vi "Dashboard Main.vi"() -> ()   [LabVIEW 2016]
uses:
  <vilib>/event_ctls.llb/eventvkey.ctl
  <vilib>/Rock Robotics/WPI/Dashboard/WPI_DashboardLogging Global.vi
  <vilib>/Utility/miscctls.llb/LVRowAndColumnTypeDef.ctl
  <vilib>/Rock Robotics/Network Tables/NT Read Numeric Array.vi
panel:
  in  "DB/Slider 0":dbl(slide) caption="Trim" scale=0.0..1.0
  in  "DB/Button 0":bool caption="Enable\nOverdrive"
  in  "DB/Slider 4":dbl(slide) caption="Aiming Aides" scale=0.0..5.0
  in  "Camera Settings Right":T1={"Frame Rate"=30, "Compression"=30, "Size"=1, "DB Camera Config"=FALSE} {"Frame Rate" scale=1.0..30.0; "Compression" scale=100.0..-1.0; "Size" items=["640x480", "320x240", "160x120"]}
  in  "Camera Name Right":string(combo)="No Camera Selection"
  out "Camera Info":cluster{"Mbps LED":bool, "Mbps":dbl, "fps":dbl} {"fps" format="%#.1g"; "Mbps" format="%#.1g"}
  in  "Camera Settings":T1={"Frame Rate"=30, "Compression"=30, "Size"=1, "DB Camera Config"=FALSE} {"Frame Rate" scale=1.0..30.0; "Compression" scale=100.0..-1.0; "Size" items=["640x480", "320x240", "160x120"]}
  in  "TCP":refnum<k5>
  in  "Rec Mode":enum32{"Stop", "Record", "Playback"}(radio)
  out "Robot IP":string
  out "Image Message":string="Timeout in Camera Communications"
  in  "Dashboard Tab":T2(tab)
  in  "Trim":dbl(slide) scale=0.0..1.0
  in  "Overdrive Enabled?":bool
  in  "Select Auto":string(combo)="Select Autonomous ..."
  out "NT Connection":bool
  out "MotorChart R":cluster{"Numeric":dbl, "Numeric":dbl}(graph)
  out "MotorChart L":cluster{"Numeric":dbl, "Numeric":dbl}(graph)
  out "MotorSliders R":cluster{"MotorSlide1":dbl, "MotorSlide2":dbl} {"MotorSlide2" scale=-1.0..1.0 scale format="%#_2e"; "MotorSlide1" scale=-1.0..1.0 scale format="%#_2e"}
  out "MotorSliders L":cluster{"MotorSlide1":dbl, "MotorSlide2":dbl} {"MotorSlide2" scale=-1.0..1.0 scale format="%#_2e"; "MotorSlide1" scale=-1.0..1.0 scale format="%#_2e"}
  out "Gyro":dbl(knob) scale=0.0..360.0
  out "JS1 Z":dbl(slide) scale=-1.0..1.0 scale format="%#_2e"
  out "JS1 Graph":cluster{"X":dbl, "Y":dbl}[](graph)
  out "JS1 Buttons":T3
  out "JS2 Z":dbl(slide) scale=-1.0..1.0 scale format="%#_2e"
  out "JS2 Graph":cluster{"X":dbl, "Y":dbl}[](graph)
  out "JS2 Buttons":T3
  out "Mode":T4(ring)=enum."Auto Disabled"
  out "Camera Image Right":T5(plugin-control)
  in  "DB/String 9":string
  in  "DB/String 8":string
  in  "DB/String 7":string
  in  "DB/String 6":string
  in  "DB/String 5":string
  in  "DB/String 4":string
  in  "DB/String 3":string
  in  "DB/String 2":string
  in  "DB/String 1":string
  in  "DB/String 0":string
  in  "DB/Slider 1":dbl(slide) caption="Aiming Aides" scale=0.0..5.0
  in  "DB/Slider 2":dbl(slide) scale=0.0..5.0
  in  "DB/Slider 3":dbl(slide) scale=0.0..5.0
  out "DB/LED 3":bool
  out "DB/LED 2":bool
  out "DB/LED 1":bool
  out "DB/LED 0":bool caption="Throttle"
  in  "DB/Button 3":bool
  in  "DB/Button 2":bool
  in  "DB/Button 1":bool
  out "Calibrated?":bool
  in  "Reset Angle":bool
  in  "Test Slider":dbl(slide) scale=0.0..100.0 scale format="%#_3g"
  in  "On/Off":bool caption="Solenoid"
  in  "Test Name":u16(ring) items=["Select the test to run..."]
  in  "Test Tree":string(tree)
  in  "Motor":cluster{"Value":dbl, "Enable":bool} {"Value" scale=-1.0..1.0 scale format="%#_3g"}
  out "Progress":T6 {"Test Progress" scale=0.0..100.0}
  in  "Rev/Fwd":cluster{"Forward":bool, "Reverse":bool}
  in  "Test Ring":u16(ring) items=["Monochrome", "Color"]
  out "Cmd Status":string
  in  "Execute Command":bool
  in  "Command Params":string[][](table)
  in  "Command Selection":i32(listbox)
  in  "CheckList":i32(listbox)
  out "Tree":string(tree)
  out "Camera Image":T5(plugin-control)
  in  "Camera Name":string(combo)="No Camera Selection"
  # "HW"
  # "HW"
  # "Joysticks"
  # "Drive Motors"
  # "Front"
  # "Right"
  # "Left"
  # "Back"
  # "This tab is a great place for autonomous settings and robot-specific values.\nPlace controls and indicators inside this tab and match name to\nDashboard Variables on robot. You can also delete this comment."
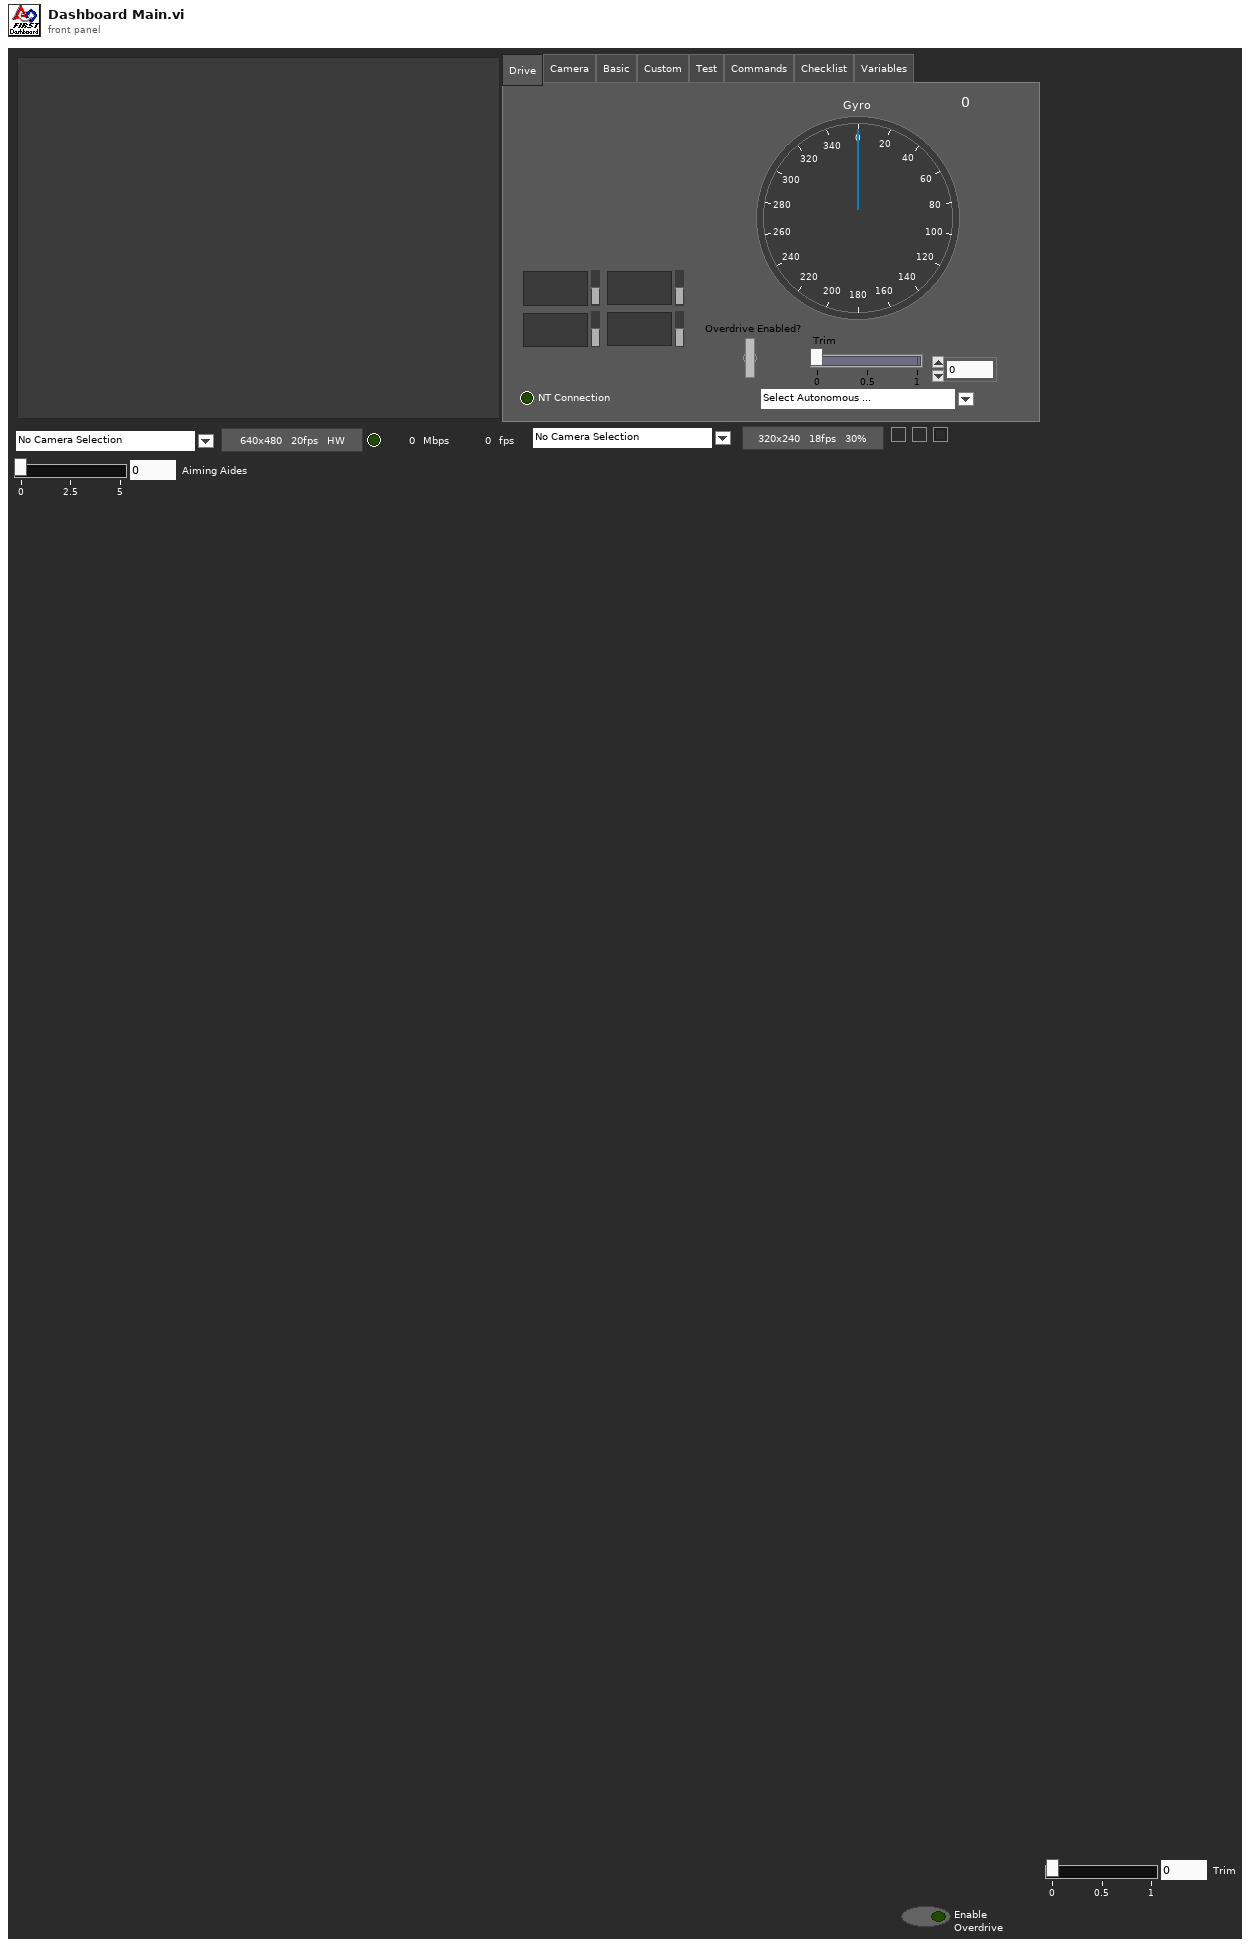
[diagram p1: front panel]
types:
  T1 = cluster{"Frame Rate":i32, "Compression":i32, "Size":u16, "DB Camera Config":bool}
  T2 = enum32{"Drive", "Camera", "Basic", "Custom", "Test", "Commands", "Checklist", "Variables"}
  T3 = cluster{bool, bool, bool, bool, bool, bool, bool, bool, bool, bool, bool, bool}
  T4 = enum8{"Tele-Op Disabled", "Tele-Op Enabled", "Auto Disabled", "Auto Enabled", "Test Disabled", "Test Enabled", "Disconnected", "No Code", "E-Stop"}
  T5 = typedef "IMAQ Image.ctl" = refnum<image>
  T6 = cluster{"Test Progress":u8, "Test Progress Text":string}
  T7 = typedef "Image Type" = u32
  T8 = cluster{"IDs":cluster{"RPC field ID":u16, "Unique ID":u16}, "String":string}
  T9 = enum32{"Drive", "Basic", "Custom", "Test", "Checklist", "Variables"}
  T10 = cluster{"Error Strings":string, "Disable Counts":cluster{u16, u16}, "Rail Faults":cluster{u16, u16, u16}, "Robot IP":string, "DB Mode":u8, "Event Info":cluster{"Name":string, "Type":u8, "Number":u16, "Replay":u8}}
  T11 = cluster{"Storage":cluster{"Disk Free":u64, "RAM Block":u32, "RAM free":u32}, "CPU Utilization":cluster{"CPU % ISR":sgl, "CPU % Time Crit":sgl, "CPU % Timed Str":sgl, "CPU % High":sgl, "CPU % Above":sgl, "CPU % Normal":sgl, "CPU % Low":sgl}, "CAN":cluster{"% Bus Utilization":sgl, "Bus Off Cnt":u32, "TX_FIFO Full Cnt":u32, "Receive Error Cnt":u8, "Transmit Error Cnt":u8}, "HID":cluster{"HID Outputs":u32, "Rumble Low":u16, "Rumble High":u16}[]}
  T12 = cluster{"Status bits":cluster{"Test Mode":bool, "Autonomous":bool, "Enabled":bool, "Code Start":bool, "Brownout":bool, "Reserved 2":bool, "Reserved 3":bool, "E-Stop":bool}, "Code Trace":cluster{"Disabled":bool, "TeleOp":bool, "Auto":bool, "Test":bool}, "Controller Type":enum16{"unknown", "cRIO", "roboRio"}, "Code?":enum16{"unknown", "noCode", "code"}, "Battery V":dbl}
  T13 = cluster{"Control Bits":cluster{"TestMode":bool, "Autonomous":bool, "Enabled":bool, "FMS Present":bool, bool, bool, bool, "E-Stop":bool}, "Team Station ":u8, "Countdown":sgl, "Joystick Values":cluster{"Axes":dbl[], "Buttons":bool[], "POVs":i16[]}[]}
  T14 = cluster{"Axes":dbl[], "Buttons":bool[], "POVs":i16[]}[]
  T15 = cluster{"Axes":dbl[], "Buttons":bool[], "POVs":i16[]}
  T16 = cluster{"Buttons[0]":bool, "Buttons[1]":bool, "Buttons[2]":bool, "Buttons[3]":bool, "Buttons[4]":bool, "Buttons[5]":bool, "Buttons[6]":bool, "Buttons[7]":bool, "Buttons[8]":bool, "Buttons[9]":bool, "Buttons[10]":bool, "Buttons[11]":bool}
  T17 = cluster{"Operation":enum16{"Update", "Clear"}, "Color Box":u32}[]
  T18 = typedef "eventvkey.ctl" = enum16{"ASCII", "Enter", "Return", "Shift", "Ctrl", "Alt", "Cmd", "Opt", "Caps", "NumLock", "Clear", "Break", "Up", "Down", "Left", "Right", "Insert", "Delete", "Home", "End", "PageUp", "PageDown", "Escape", "Help", "Pause", "ScrollLock", "F1", "F2", "F3", "F4", "F5", "F6", "F7", "F8", "F9", "F10", "F11", "F12", "F13", "F14", "F15", "F16", "F17", "F18", "F19", "F20", "F21", "F22", "F23", "F24", "Play", "VolumeUp", "VolumeDown", "Mute", "Two Byte Char"}
  T19 = cluster{"Image Size":bool, "Image Type":bool, "Pixel Value":bool, "ROI Information":bool, "Zoom Factor":bool}
  T20 = cluster{"Operation":enum16{"Update", "Clear"}, "Color Box":u32}
  T21 = typedef "LVRowAndColumnTypeDef.ctl" = cluster{"Row":i32, "Column":i32}
  T22 = cluster{"Shift":bool, "Ctrl":bool, "Alt":bool, "Cmd":bool, "Opt":bool}
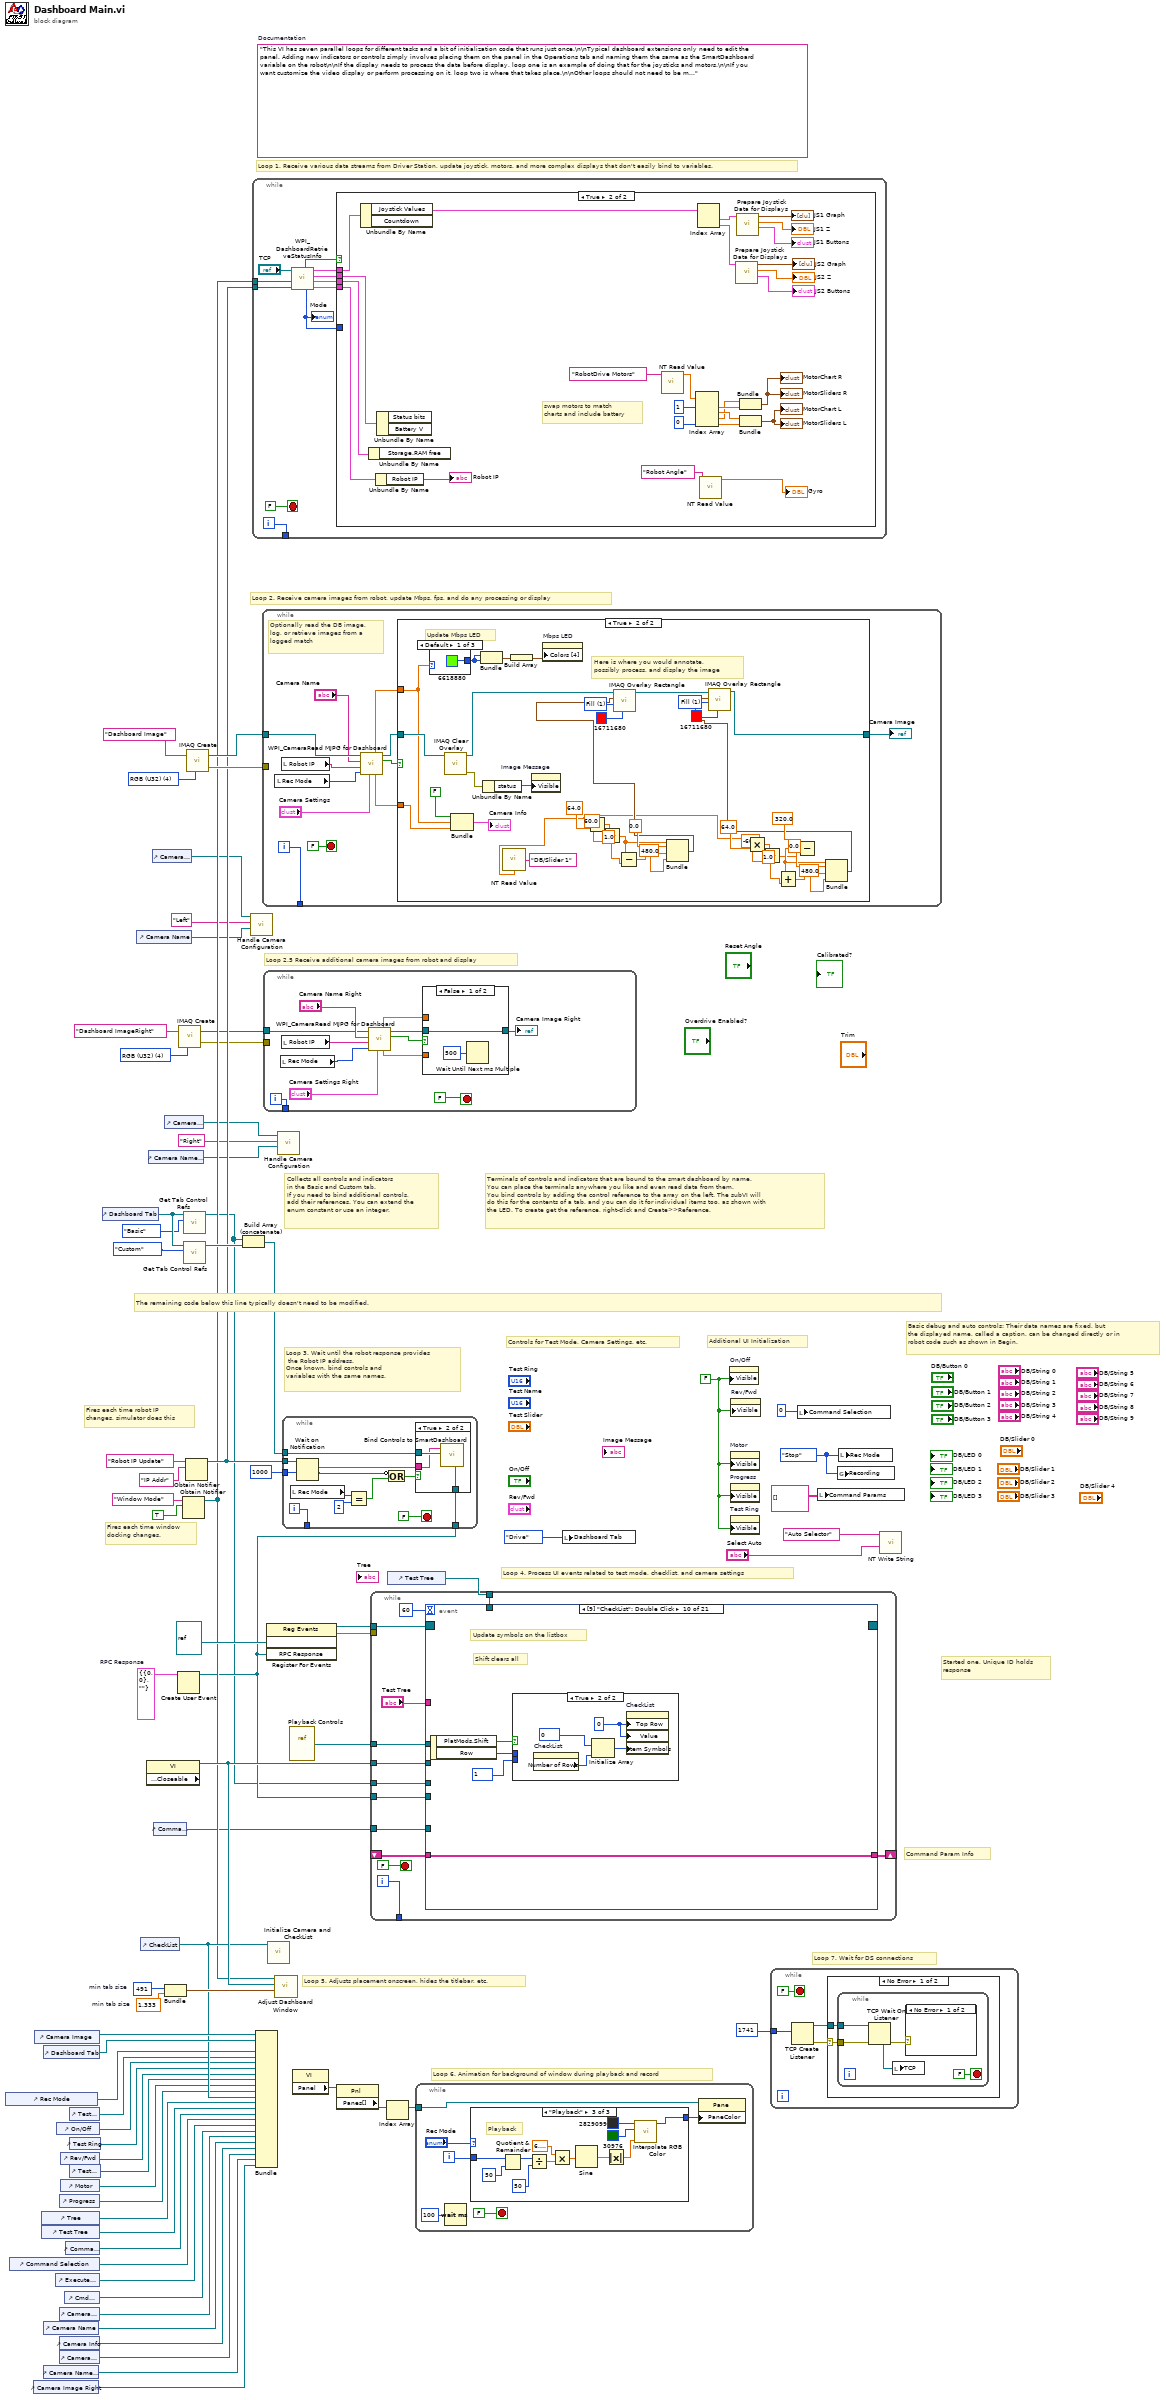
[diagram p0: block diagram]
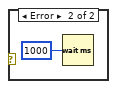
[diagram p3: hidden frame]
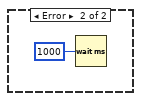
[diagram p4: hidden frame]
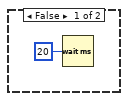
[diagram p5: hidden frame]
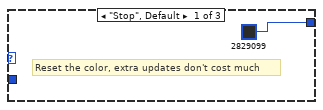
[diagram p6: hidden frame]
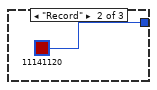
[diagram p7: hidden frame]
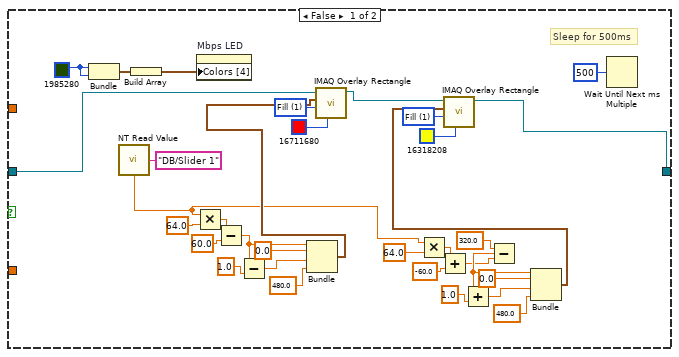
[diagram p9: hidden frame]
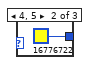
[diagram p10: hidden frame]
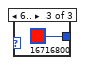
[diagram p11: hidden frame]
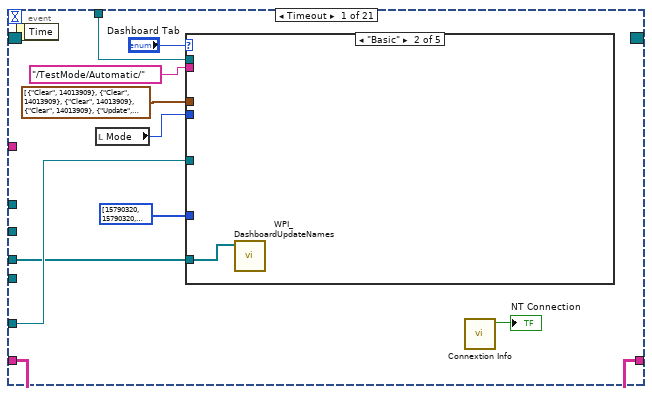
[diagram p12: hidden frame]
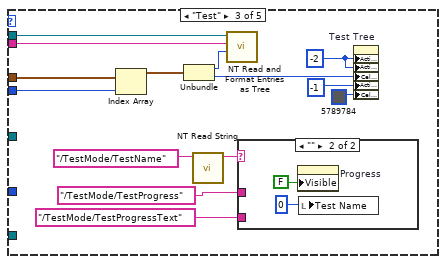
[diagram p14: hidden frame]
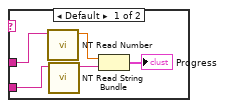
[diagram p15: hidden frame]
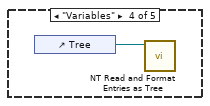
[diagram p16: hidden frame]
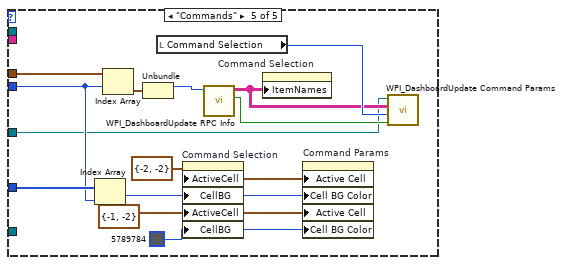
[diagram p17: hidden frame]
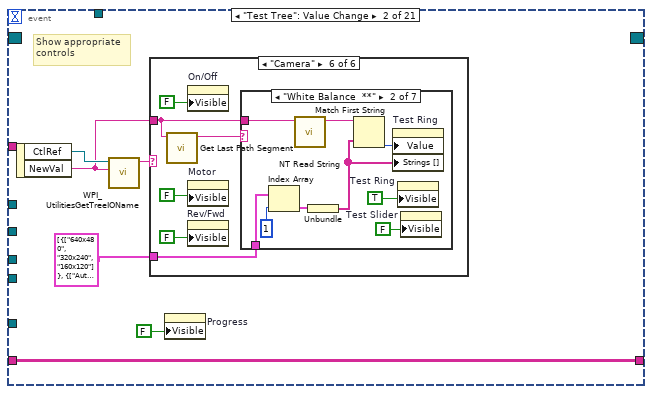
[diagram p18: hidden frame]
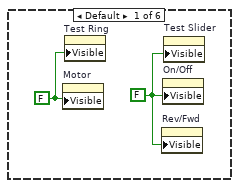
[diagram p19: hidden frame]
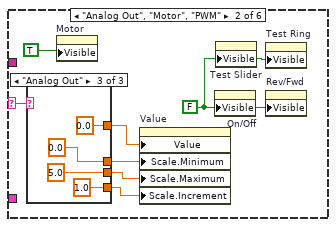
[diagram p20: hidden frame]
diagram:
  w10 = T7 4 items=["Grayscale (U8)", "Grayscale (I16)", "Grayscale (SGL)", "Complex (CSG)", "RGB (U32)", "HSL (U32)", "RGB (U64)"] ("Image Type")
  w26 = T8 {"IDs"={"RPC field ID"=0, "Unique ID"=0}, "String"=""}  # RPC Response
  w49 = 491  # min tab size
  w48 = 1.333  # min tab size
  w56 = enum32{"Stop", "Record", "Playback"}."Stop" ("Rec Mode")
  w33 = FALSE ("Visible")
  (unwired) "This VI has seven parallel loops for different tasks and a bit of initialization code that runs just once.\n\nTypical dashboard extensions only need to edit the panel. Adding new indicators or controls simply involves placing them on the panel in the Operations tab and naming them the same as the SmartDashboard variable on the robot\n\nIf the display needs to process the data before display, loop one is an example of doing that for the joysticks and motors.\n\nIf you want customize the video display or perform processing on it, loop two is where that takes place.\n\nOther loops should not need to be modified. They are pretty standard, and document the task they perform."  # Documentation
  w73 = T7 4 items=["Grayscale (U8)", "Grayscale (I16)", "Grayscale (SGL)", "Complex (CSG)", "RGB (U32)", "HSL (U32)", "RGB (U64)"] ("Image Type")
  # "Loop 2.5 Receive additional camera images from robot and display"
  # "Command Param Info"
  # "Started one, Unique ID holds\nresponse"
  # "Loop 7. Wait for DS connections"
  # "Basic debug and auto controls: Their data names are fixed, but\nthe displayed name, called a caption, can be changed directly or in\nrobot code such as shown in Begin."
  # "Controls for Test Mode, Camera Settings, etc."
  # "Additional UI Initialization"
  # "Loop 6. Animation for background of window during playback and record"
  # "Fires each time robot IP\nchanges, simulator does this"
  # "Fires each time window\ndocking changes."
  # "Collects all controls and indicators\nin the Basic and Custom tab.\nIf you need to bind additional controls,\nadd their references. You can extend the\nenum constant or use an integer."
  # "The remaining code below this line typically doesn't need to be modified."
  # "Loop 4. Process UI events related to test mode, checklist, and camera settings"
  # "Terminals of controls and indicators that are bound to the smart dashboard by name.\nYou can place the terminals anywhere you like and even read data from them.\nYou bind controls by adding the control reference to the array on the left. The subVI will\ndo this for the contents of a tab, and you can do it for individual items too, as shown with\nthe LED. To create get the reference, right-click and Create>>Reference."
  # "Loop 3. Wait until the robot response provides\n the Robot IP address.\nOnce known, bind controls and\nvariables with the same names."
  # "Loop 5. Adjusts placement onscreen, hides the titlebar, etc."
  # "Loop 1. Receive various data streams from Driver Station, update joystick, motors, and more complex displays that don't easily bind to variables."
  # "Loop 2. Receive camera images from robot, update Mbps, fps, and do any processing or display"
  n1 = control-ref of="Rec Mode"() -> (w39:refnum<vi>)
  n2 = control-ref of="Command Selection"() -> (w25:refnum<vi>)
  n3 = control-ref of="Camera Image Right"() -> (w1:refnum<vi>)
  n4 = control-ref of="Camera Image"() -> (w51:refnum<vi>)
  n5 = control-ref of="Tree"() -> (w43:refnum<vi>)
  n6 = control-ref of="Test Tree"() -> (w42:refnum<vi>)
  n7 = control-ref of="Dashboard Tab"() -> (w50:refnum<vi>)
  n8 = control-ref of="Camera Name"() -> (w16:refnum<vi>)
  n9 = control-ref of="Camera Name Right"() -> (w2:refnum<vi>)
  n10 = control-ref of="Execute Command"() -> (w27:refnum<vi>)
  n11 = control-ref of="On/Off"() -> (w37:refnum<vi>)
  n12 = control-ref of="Progress"() -> (w34:refnum<vi>)
  n13 = control-ref of="Camera Settings"() -> (w17:refnum<vi>)
  n14 = control-ref of="Camera Info"() -> (w15:refnum<vi>)
  n15 = control-ref of="Camera Settings Right"() -> (w3:refnum<vi>)
  n16 = control-ref of="Rev/Fwd"() -> (w35:refnum<vi>)
  n17 = control-ref of="Motor"() -> (w40:refnum<vi>)
  n18 = control-ref of="Cmd Status"() -> (w21:refnum<vi>)
  n19 = control-ref of="Command Params"() -> (w28:refnum<vi>)
  n20 = control-ref of="Test Slider"() -> (w38:refnum<vi>)
  n21 = control-ref of="Test Ring"() -> (w36:refnum<vi>)
  n22 = control-ref of="Test Name"() -> (w41:refnum<vi>)
  n23 = control-ref of="Dashboard Tab"() -> (w54:refnum<vi>)
  n24 = control-ref of="Camera Name"() -> (w18:refnum<vi>)
  n25 = control-ref of="CheckList"() -> (w44:refnum<vi>)
  n26 = property class="VI" props=["Front Panel.Closeable"]() -> (reference out=w55:refnum<vi>)  [unwired: 2 in, 2 out]
  n27 = control-ref of="Camera Name Right"() -> (w6:refnum<vi>)
  n28 = control-ref of="Camera Settings"() -> (w19:refnum<vi>)
  n29 = control-ref of="Command Params"() -> (w20:refnum<vi>)
  n30 = control-ref of="Camera Settings Right"() -> (w7:refnum<vi>)
  n31 = Bundle("min tab size"=w49, "min tab size"=w48) -> (w47:cluster{"min tab size":i32, "min tab size":dbl})  [unwired: 1 in]
  n32 = Create User Event(user event datatype=w26) -> (user event=w22:refnum<user-event>)  [unwired: 1 in, 1 out]
  n33 = call "IMAQ Create"("Image Name"="Dashboard ImageRight", "Image Type"=w10) -> ("New Image"=w9:T5, "error out"=w8:errorcluster)  [unwired: 2 in, 1 out]
  n34 = Obtain Notifier(name (unnamed)="Window Mode", notification data type=TRUE) -> (notifier out=w31:refnum<notifier>)  [unwired: 2 in, 2 out]
  n35 = call <vilib>:"Get Tab Control Refs.vi"("Page Index"=T9."Basic" ("Dashboard Tab"), "TabControl in"=w54) -> ("ControlsOnPage"=w14:refnum<vi>[])  [unwired: 9 in]
  n36 = call <vilib>:"Get Tab Control Refs.vi"("Page Index"=T9."Custom" ("Dashboard Tab"), "TabControl in"=w54) -> ("ControlsOnPage"=w53:refnum<vi>[])  [unwired: 9 in]
  n37 = Obtain Notifier(name (unnamed)="Robot IP Update", notification data type="IP Addr" ("name (unnamed)")) -> (notifier out=w32:refnum<notifier>)  [unwired: 2 in, 2 out]
  n38 = call "IMAQ Create"("Image Name"="Dashboard Image", "Image Type"=w73) -> ("New Image"=w71:T5, "error out"=w70:errorcluster)  [unwired: 2 in, 1 out]
  n39 = Build Array (concatenate)(w14, w53) -> (w52:refnum<vi>[])
  n40 = call "Handle Camera Configuration.vi"("CameraNameRef"=w18, "Camera File Name"="Left", "ClusterRef"=w19) -> ()  [unwired: 9 in]
  n41 = while {
    tunnel: [w83] -> _
    tunnel: w32 -> [w77]
    tunnel: w31 -> [w74]
    i -> [w83]
    stop <- FALSE stop-if-true
    n42 = call <vilib>:"WPI_DashboardRetrieveStatusInfo.vi"("Binding Refnum"=w77, "Window Mode Notifier"=w74, "TCP Cnx"="TCP") -> ("Power and Errors"=w78:T10, "Robot Metrics"=w81:T11, "Status Info"=w82:T12, "Control Info"=w79:T13, "Robot Mode"=w76:T4, "Process?"=w80:bool)  [unwired: 3 in]
    "Mode" <- w76
    n43 = case shown="True" w80 {
      tunnel: w82 -> [_ w111]
      tunnel: w81 -> [_ w110]
      tunnel: w79 -> [_ w109]
      tunnel: w78 -> [_ w108]
      tunnel: w76 -> [_ _]
      frame False {
        n44 = Wait (ms)(milliseconds to wait=u32 20) -> ()  [unwired: 1 out]
      }
      frame True {
        # "swap motors to match\ncharts and include battery"
        n45 = Unbundle By Name(w109) -> ("Joystick Values"=w99:T14)  [unwired: 1 out]
        n46 = Unbundle By Name(w110) -> ()  [unwired: 1 out]
        n47 = Unbundle By Name(w108) -> ("Robot IP"=→"Robot IP":string)
        n48 = Unbundle By Name(w111) -> ()  [unwired: 2 out]
        n49 = call-poly <vilib>:"NT Read Value.vi"("Name"="RobotDrive Motors") -> ("Numeric Array"=w89:dbl[])  [unwired: 9 in, 1 out]
        n50 = Index Array(array=w89, index #1=1, index #4=0) -> (element #1=w103:dbl, element #2=w104:dbl, element #3=w102:dbl, element #4=w107:dbl)  [unwired: 2 in]
        n51 = Index Array(array=w99) -> (element #1=w98:T15, element #2=w94:T15)  [unwired: 2 in]
        n52 = call-poly <vilib>:"NT Read Value.vi"("Name"="Robot Angle") -> ("Numeric"=→"Gyro":dbl)  [unwired: 9 in, 1 out]
        n53 = call "Prepare Joystick Data for Displays.vi"("Joystick Values"=w94) -> ("Buttons"=→"JS2 Buttons":T16, "Z Axis"=→"JS2 Z":dbl, "Cartesian Data"=→"JS2 Graph":cluster{"X axis":dbl, "X axis":dbl}[])  [unwired: 8 in]
        n54 = call "Prepare Joystick Data for Displays.vi"("Joystick Values"=w98) -> ("Buttons"=→"JS1 Buttons":T16, "Z Axis"=→"JS1 Z":dbl, "Cartesian Data"=→"JS1 Graph":cluster{"X axis":dbl, "X axis":dbl}[])  [unwired: 8 in]
        n55 = Bundle("Numeric"=w102, "Numeric"=w103) -> (→"MotorChart R" →"MotorSliders R":cluster{"Numeric":dbl, "Numeric":dbl})  [unwired: 1 in]
        n56 = Bundle("Numeric"=w104, "Numeric"=w107) -> (→"MotorChart L" →"MotorSliders L":cluster{"Numeric":dbl, "Numeric":dbl})  [unwired: 1 in]
      }
    }
  }
  n57 = Bundle("Camera Image"=w51, "Dashboard Tab"=w50, "Rec Mode"=w39, "Test Slider"=w38, "On/Off"=w37, "Test Ring"=w36, "Rev/Fwd"=w35, "Test Name"=w41, "Motor"=w40, "Progress"=w34, "CheckList"=w44, "Tree"=w43, "Test Tree"=w42, "Command Params"=w28, "Command Selection"=w25, "Execute Command"=w27, "Cmd Status"=w21, "Camera Settings"=w17, "Camera Name"=w16, "Camera Info"=w15, "Camera Settings Right"=w3, "Camera Name Right"=w2, "Camera Image Right"=w1) -> ()  [unwired: 2 in, 1 out]
  n58 = while {
    tunnel: w71 -> [w121]
    tunnel: w70 -> [_]
    tunnel: [w122] -> _
    i -> [w122]
    stop <- FALSE stop-if-true
    # "Optionally read the DB image,\nlog, or retrieve images from a\nlogged match"
    n59 = local read "Rec Mode"() -> (w117:enum32{"Stop", "Record", "Playback"})
    n60 = local read "Robot IP"() -> (w116:string)
    n61 = call <vilib>:"WPI_CameraRead MJPG for Dashboard.vi"("Camera Settings"="Camera Settings", "Rec Mode"=w117, "Robot IP"=w116, "Camera Name"="Camera Name", "Refnum in"=w121) -> ("Active"=w119:bool, "Refnum out"=w120:T5, "FPS"=w118:dbl, "Bandwidth (Mbps)"=w115:dbl)  [unwired: 3 in]
    n62 = case shown="True" w119 {
      tunnel: w120 -> [w144 w191]
      tunnel: w115 -> [_ w188]
      tunnel: w118 -> [_ w189]
      tunnel: [w131 w183] -> w112
      frame False {
        w129 = u32 1 items=["Frame", "Fill", "Highlight"] ("Drawing Mode (Frame)")
        w147 = u32 1 items=["Frame", "Fill", "Highlight"] ("Drawing Mode (Frame)")
        w154 = u32 1985280 ("Color Box")
        # "Sleep for 500ms"
        n63 = Bundle("Color Box"=w154, "Color Box"=w154) -> (w155:cluster{"Color Box":u32, "Color Box":u32})  [unwired: 1 out]
        n64 = call-poly <vilib>:"NT Read Value.vi"("Name"="DB/Slider 1") -> ("Numeric"=w127:dbl)  [unwired: 9 in, 1 out]
        n65 = Build Array(w155) -> (w153:cluster{"Color Box":u32, "Color Box":u32}[])
        n66 = Multiply(x=w127, y=64.0) -> (x*y=w142:dbl)
        n67 = property on="Mbps LED" class="Bool (strict)"("Colors [4]"=w153) -> ()  [unwired: 2 in, 2 out]
        n68 = Subtract(x=w142, y=60.0) -> (x-y=w143:dbl)
        n69 = Subtract(x=w143, y=1.0) -> (x-y=w140:dbl)
        n70 = Bundle(w143, 0.0, w140, 480.0) -> (w145:cluster{dbl, dbl, dbl, dbl})  [unwired: 1 in]
        n71 = call "IMAQ Overlay Rectangle"("Color"=u32 16711680, "Drawing Mode (Frame)"=w147, "Rectangle"=w145, "Image"=w144) -> ("Image Out"=w132:T5)  [unwired: 6 in, 1 out]
        n72 = Multiply(x=w127, y=64.0) -> (x*y=w136:dbl)
        n73 = Add(x=w136, y=-60.0) -> (x+y=w124:dbl)
        n74 = Subtract(x=320.0, y=w124) -> (x-y=w125:dbl)
        n75 = Add(x=w125, y=1.0) -> (x+y=w134:dbl)
        n76 = Bundle(w125, 0.0, w134, 480.0) -> (w130:cluster{dbl, dbl, dbl, dbl})  [unwired: 1 in]
        n77 = call "IMAQ Overlay Rectangle"("Color"=u32 16318208, "Drawing Mode (Frame)"=w129, "Rectangle"=w130, "Image"=w132) -> ("Image Out"=w131:T5)  [unwired: 6 in, 1 out]
        n78 = Wait Until Next ms Multiple(millisecond multiple=u32 500) -> ()  [unwired: 1 out]
      }
      frame True {
        w160 = u32 1 items=["Frame", "Fill", "Highlight"] ("Drawing Mode (Frame)")
        w182 = u32 1 items=["Frame", "Fill", "Highlight"] ("Drawing Mode (Frame)")
        # "Here is where you would annotate,\npossibly process, and display the image"
        # "Update Mbps LED"
        n79 = case shown="Default" w188 {
          tunnel: [u32 6618880 ("Color Box") u32 16776722 ("Color Box") u32 16716800 ("Color Box")] -> w192
          frame Default {
          }
          frame 4, 5 {
          }
          frame 6.. {
          }
        }
        n80 = call "IMAQ Clear Overlay"("Image"=w191) -> ("error out"=w194:errorcluster, "Image Out"=w185:T5)  [unwired: 2 in, 7 out]
        n81 = Bundle(FALSE, "Bandwidth (Mbps)"=w188, "FPS"=w189) -> (→"Camera Info":cluster{bool, "Bandwidth (Mbps)":dbl, "FPS":dbl})  [unwired: 1 in]
        n82 = Bundle("Color Box"=w192, "Color Box"=w192) -> (w193:cluster{"Color Box":u32, "Color Box":u32})  [unwired: 1 out]
        n83 = Unbundle By Name(w194) -> ("status"=w195:bool)
        n84 = call-poly <vilib>:"NT Read Value.vi"("Name"="DB/Slider 1") -> ("Numeric"=w157:dbl)  [unwired: 9 in, 1 out]
        n85 = Build Array(w193) -> (w190:cluster{"Color Box":u32, "Color Box":u32}[])
        n86 = property on="Image Message" class="Str"("Visible"=w195) -> ()  [unwired: 2 in, 2 out]
        n87 = property on="Mbps LED" class="Bool (strict)"("Colors [4]"=w190) -> ()  [unwired: 2 in, 2 out]
        n88 = Multiply(x=w157, y=64.0) -> (x*y=w175:dbl)
        n89 = Subtract(x=w175, y=60.0) -> (x-y=w176:dbl)
        n90 = Subtract(x=w176, y=1.0) -> (x-y=w173:dbl)
        n91 = Bundle(w176, 0.0, w173, 480.0) -> (w162:cluster{dbl, dbl, dbl, dbl})  [unwired: 1 in]
        n92 = call "IMAQ Overlay Rectangle"("Color"=u32 16711680, "Drawing Mode (Frame)"=w182, "Rectangle"=w162, "Image"=w185) -> ("Image Out"=w184:T5)  [unwired: 6 in, 1 out]
        n93 = Multiply(x=w157, y=64.0) -> (x*y=w169:dbl)
        n94 = Add(x=w169, y=-60.0) -> (x+y=w163:dbl)
        n95 = Subtract(x=320.0, y=w163) -> (x-y=w164:dbl)
        n96 = Add(x=w164, y=1.0) -> (x+y=w167:dbl)
        n97 = Bundle(w164, 0.0, w167, 480.0) -> (w161:cluster{dbl, dbl, dbl, dbl})  [unwired: 1 in]
        n98 = call "IMAQ Overlay Rectangle"("Color"=u32 16711680, "Drawing Mode (Frame)"=w160, "Rectangle"=w161, "Image"=w184) -> ("Image Out"=w183:T5)  [unwired: 6 in, 1 out]
      }
    }
    "Camera Image" <- w112
  }
  n99 = while {
    tunnel: w9 -> [w209]
    tunnel: w8 -> [_]
    tunnel: [w203] -> _
    i -> [w203]
    stop <- FALSE stop-if-true
    n100 = local read "Rec Mode"() -> (w207:enum32{"Stop", "Record", "Playback"})
    n101 = local read "Robot IP"() -> (w208:string)
    n102 = call <vilib>:"WPI_CameraRead MJPG for Dashboard.vi"("Camera Settings"="Camera Settings Right", "Rec Mode"=w207, "Robot IP"=w208, "Camera Name"="Camera Name Right", "Refnum in"=w209) -> ("Active"=w202:bool, "Refnum out"=w205:T5, "FPS"=w200:dbl, "Bandwidth (Mbps)"=w201:dbl)  [unwired: 3 in]
    n103 = case shown="False" w202 {
      tunnel: w205 -> [w211 w213]
      tunnel: w201 -> [_ _]
      tunnel: w200 -> [_ _]
      tunnel: [w211 w213] -> w199
      frame False {
        n104 = Wait Until Next ms Multiple(millisecond multiple=u32 500) -> ()  [unwired: 1 out]
      }
      frame True {
      }
    }
    "Camera Image Right" <- w199
  }
  n105 = register-events(refnum<vi> refnum, w22) -> (reference out=w60:refnum<event-registration>, error out=w59:errorcluster)  [unwired: 2 in]
  n106 = call "Initialize Camera and CheckList.vi"("ListBox in"=w44) -> ()  [unwired: 11 in]
  n107 = call "Adjust Dashboard Window.vi"("Size Constraints"=w47, "VI"=w55, "WIn Mode"=w31) -> ()  [unwired: 9 in]
  n108 = call "Handle Camera Configuration.vi"("CameraNameRef"=w6, "Camera File Name"="Right", "ClusterRef"=w7) -> ()  [unwired: 9 in]
  n109 = while {
    tunnel: w52 -> [w225]
    tunnel: w32 -> [w223]
    tunnel: [w221] -> _
    tunnel: u32 1000 ("milliseconds to wait") -> [w220]
    tunnel: w22 -> [w214]
    i -> [w221]
    stop <- FALSE stop-if-true
    n110 = local read "Rec Mode"() -> (w216:enum32{"Stop", "Record", "Playback"})
    n111 = Wait on Notification(notifier=w223, timeout in ms (-1)=w220) -> (notification=w222:string, timed out?=w218:bool)  [unwired: 2 in, 2 out]
    n112 = Equal?(x=w216, y=u16 2 ("Rec Mode")) -> (x = y?=w217:bool)
    n113 = Compound Arithmetic op=OR(invert w218, w217) -> (w219:bool)
    n114 = case shown="True" w219 {
      tunnel: w225 -> [_ w228]
      tunnel: w222 -> [_ w227]
      tunnel: w214 -> [_ w226]
      frame False {
      }
      frame True {
        n115 = call <vilib>:"Bind Controls to SmartDashboard.vi"("RPC ref"=w226, "Bound Control Refs"=w228, "Server IP Address"=w227) -> ()  [unwired: 9 in]
      }
    }
  }
  n116 = vi-ref "Playback Controls.vi"() -> (w61:refnum<vi>)
  n117 = property class="VI"() -> ("Panel"=w63:refnum<vi>)  [unwired: 2 in, 2 out]
  n118 = property class="Pnl"(reference=w63) -> ("Panes[]"=w64:refnum<vi>[])  [unwired: 1 in, 2 out]
  n119 = Index Array(array=w64) -> (element=w62:refnum<vi>)  [unwired: 1 in]
  n120 = control-ref of="Test Tree"() -> (w65:refnum<vi>)
  n121 = while {
    tunnel: [w238] -> _
    tunnel: w65 -> [w237]
    tunnel: w61 -> [w236]
    tunnel: w60 -> [w235]
    tunnel: w59 -> [_]
    tunnel: w55 -> [w234]
    tunnel: w22 -> [w233]
    tunnel: w20 -> [w232]
    shift-right: [w231] -> _
    shift-left: _ -> [w230]
    tunnel: w14 -> [w229]
    i -> [w238]
    stop <- FALSE stop-if-true
    n122 = event shown="[9] \"CheckList\": Double Click" {
      selector: w235 -> [_ _ _ _ _ _ _ _ _ _ _ _ _ _ _ _ _ _ _ _ _]
      dyn-events: [_ _ _ _ _ _ _ _ _ _ _ _ _ _ _ _ w494 _ _ _ _] -> _
      timeout: u32 60 ("milliseconds to wait") -> [_ _ _ _ _ _ _ _ _ _ _ _ _ _ _ _ _ _ _ _ _]
      tunnel: w237 -> [w250 _ _ _ _ _ _ _ _ _ _ _ _ _ _ _ _ _ _ _ _]
      tunnel: "Test Tree" -> [_ _ _ _ _ _ _ _ _ _ _ w461 w469 w471 w475 w483 _ _ _ _ _]
      tunnel: w236 -> [_ _ _ _ _ _ _ _ _ _ _ _ _ _ _ _ w496 _ w514 _ _]
      tunnel: w234 -> [_ _ _ _ _ _ _ _ _ _ _ _ _ _ _ _ w492 _ _ _ _]
      tunnel: w233 -> [_ _ _ _ _ _ _ _ _ _ _ _ _ _ _ _ w488 _ _ _ _]
      tunnel: w232 -> [w245 _ _ _ _ _ w412 _ _ _ _ _ _ _ _ _ _ _ _ _ _]
      tunnel: [w244 w289 w391 w396 w405 w409 w410 w419 w429 w436 w448 w460 w467 w470 w474 w482 w487 w509 w511 w515 w526] -> w231
      tunnel: w230 -> [w244 w289 w391 w396 w405 w409 w410 _ _ w436 w448 w460 w467 w470 w474 w482 w487 w509 w511 w515 w526]
      tunnel: w229 -> [w242 _ _ _ _ _ _ _ _ _ _ _ _ _ _ _ _ _ _ _ _]
      event Timeout {
        n123 = event-data() -> ()  [unwired: 1 in, 1 out]
        n124 = local read "Mode"() -> (w247:T4)
        n125 = case shown="\"Basic\"" "Dashboard Tab" {
          tunnel: w250 -> [_ _ w266 _ _]
          tunnel: "/TestMode/Automatic/" ("Name Pattern") -> [_ _ w265 _ _]
          tunnel: T17 [{"Operation"=enum."Clear", "Color Box"=14013909}, {"Operation"=enum."Clear", "Color Box"=14013909}, {"Operation"=enum."Clear", "Color Box"=14013909}, {"Operation"=enum."Clear", "Color Box"=14013909}, {"Operation"=enum."Update", "Color Box"=14013909}, {"Operation"=enum."Update", "Color Box"=16777215}, {"Operation"=enum."Clear", "Color Box"=14013909}, {"Operation"=enum."Clear", "Color Box"=14013909}, {"Operation"=enum."Clear", "Color Box"=14013909}] -> [_ _ w258 _ w282]
          tunnel: w247 -> [_ _ w257 _ w281]
          tunnel: u32[] [15790320, 15790320, 15790320, 15790320, 16777215, 16777215, 15790320, 15790320, 15790320] -> [_ _ _ _ w287]
          tunnel: w245 -> [_ _ _ _ w275]
          tunnel: w242 -> [_ w252 _ _ _]
          frame "Custom", Default {
          }
          frame "Basic" {
            n126 = call <vilib>:"WPI_DashboardUpdateNames.vi"("Controls on Tab"=w252) -> ()  [unwired: 11 in]
          }
          frame "Test" {
            w264 = -2 ("Active Item:Row Number")
            n127 = Index Array(array=w258, index=w257) -> (element=w259:T20)
            n128 = Unbundle(w259) -> ("Operation"=w260:enum16{"Update", "Clear"}, "Color Box"=w261:u32)
            n129 = call <vilib>:"NT Read String.vi"("Name"="/TestMode/TestName") -> ("String"=w255:string)  [unwired: 9 in, 1 out]
            n130 = call <vilib>:"NT Read and Format Entries as Tree.vi"("Operation"=w260, "Name Pattern"=w265, "Tree Refnum"=w266) -> ()  [unwired: 7 in, 2 out]
            n131 = case shown="\"\"" w255 {
              tunnel: "/TestMode/TestProgress" ("Name") -> [w268 _]
              tunnel: "/TestMode/TestProgressText" ("Name") -> [w267 _]
              frame Default {
                n132 = call <vilib>:"NT Read Number.vi"("Name"=w268) -> ("Numeric"=w269:dbl)  [unwired: 9 in, 1 out]
                n133 = call <vilib>:"NT Read String.vi"("Name"=w267) -> ("String"=w270:string)  [unwired: 9 in, 1 out]
                n134 = Bundle("Numeric"=w269, "String"=w270) -> (→"Progress":cluster{"Numeric":dbl, "String":string})  [unwired: 1 in]
              }
              frame "" {
                n135 = property on="Progress" class="Clust (strict)"("Visible"=FALSE) -> ()  [unwired: 2 in, 2 out]
                n136 = local write "Test Name"(u16 0) -> ()
              }
            }
            n137 = property on="Test Tree" class="Tree (strict)"("Active Item Row Number"=w264, "ActiveColNum"=w264, "CellBG"=w261, "Active Item Row Number"=-1 ("Active Item:Row Number"), "CellBG"=u32 5789784 ("Color Box")) -> ()  [unwired: 2 in, 2 out]
          }
          frame "Variables" {
            n138 = control-ref of="Tree"() -> (w274:refnum<vi>)
            n139 = call <vilib>:"NT Read and Format Entries as Tree.vi"("Tree Refnum"=w274) -> ()  [unwired: 9 in, 2 out]
          }
          frame "Commands" {
            w283 = u32 5789784 ("Color Box")
            w284 = T21 {"Row"=-1, "Column"=-2} ("Active Cell:Active Cell")
            w286 = T21 {"Row"=-2, "Column"=-2} ("Active Cell:Active Cell")
            n140 = Index Array(array=w287, index=w281) -> (element=w285:u32)
            n141 = Index Array(array=w282, index=w281) -> (element=w280:T20)
            n142 = Unbundle(w280) -> ("Operation"=w279:enum16{"Update", "Clear"})  [unwired: 1 out]
            n143 = local read "Command Selection"() -> (w278:i32)
            n144 = property on="Command Selection" class="MCListbox (strict)"("ActiveCell"=w286, "CellBG"=w285, "ActiveCell"=w284, "CellBG"=w283) -> ()  [unwired: 2 in, 2 out]
            n145 = call <vilib>:"WPI_DashboardUpdate RPC Info.vi"("Operation"=w279) -> ("update"=w277:bool, "commands"=w276:string[][])  [unwired: 9 in]
            n146 = property on="Command Selection" class="MCListbox (strict)"("ItemNames"=w276) -> ()  [unwired: 2 in, 2 out]
            n147 = property on="Command Params" class="Tbl (strict)"("Active Cell"=w286, "Cell BG Color"=w285, "Active Cell"=w284, "Cell BG Color"=w283) -> ()  [unwired: 2 in, 2 out]
            n148 = call <vilib>:"WPI_DashboardUpdate Command Params.vi"("Update"=w277, "NewVal"=w278, "Commands"=w276, "Param Tbl"=w275) -> ()  [unwired: 7 in, 1 out]
          }
        }
        n149 = call <vilib>:"Connextion Info.vi"() -> ("Connected"=→"NT Connection":bool)  [unwired: 10 in, 1 out]
      }
      event "Test Tree": Value Change {
        # "Show appropriate\ncontrols"
        n150 = event-data() -> ("CtlRef"=w292:refnum<vi>, "NewVal"=w290:string)  [unwired: 1 in]
        n151 = call <vilib>:"WPI_UtilitiesGetTreeIOName.vi"("NewVal"=w290, "TreeControl in"=w292) -> ("I/O Name"=w293:string)  [unwired: 9 in]
        n152 = case shown="\"Camera\"" w293 {
          selector: w293 -> [_ w300 _ w322 w331 _]
          tunnel: w290 -> [_ _ w319 w321 _ w338]
          tunnel: cluster{string[]}[] [{["640x480", "320x240", "160x120"]}, {["Auto", "Fixed indoor", "Fixed outdoor 1", "Fixed outdoor 2", "Fixed fluorescent 1", "Fixed fluorescent 2", "Hold current"]}, {["Auto", "Flicker-free 50 Hz", "Flicker-free 60 Hz", "Hold current"]}, {["None", "Prioritize frame rate", "Prioritize image quality"]}, {["Monochrome", "Color"]}] -> [_ _ _ _ _ w337]
          frame Default {
            w295 = FALSE ("Visible")
            w294 = FALSE ("Visible")
            n153 = property on="Motor" class="Clust (strict)"("Visible"=w294) -> ()  [unwired: 2 in, 2 out]
            n154 = property on="Test Ring" class="Ring (strict)"("Visible"=w294) -> ()  [unwired: 2 in, 2 out]
            n155 = property on="Rev/Fwd" class="Clust (strict)"("Visible"=w295) -> ()  [unwired: 2 in, 2 out]
            n156 = property on="On/Off" class="Bool (strict)"("Visible"=w295) -> ()  [unwired: 2 in, 2 out]
            n157 = property on="Test Slider" class="Slide (strict)"("Visible"=w295) -> ()  [unwired: 2 in, 2 out]
          }
          frame "Analog Out", "Motor", "PWM" {
            w301 = FALSE ("Visible")
            n158 = case shown="\"Analog Out\"" w300 {
              tunnel: [1.0 ("Value") -1.0 ("Value") 0.0 ("Value")] -> w299
              tunnel: [255.0 ("Value") 1.0 ("Value") 5.0 ("Value")] -> w298
              tunnel: [128.0 ("Value") 0.0 ("Value") 0.0 ("Value")] -> w297
              tunnel: [64.0 ("Value") 0.5 ("Value") 1.0 ("Value")] -> w296
              frame "PWM" {
              }
              frame "Motor", Default {
              }
              frame "Analog Out" {
              }
            }
            n159 = property on="Motor" class="Clust (strict)"("Visible"=TRUE) -> ()  [unwired: 2 in, 2 out]
            n160 = property on="Value" class="Slide (strict)"("Value"=w297, "Scale.Minimum"=w299, "Scale.Maximum"=w298, "Scale.Increment"=w296) -> ()  [unwired: 2 in, 2 out]
            n161 = property on="On/Off" class="Bool (strict)"("Visible"=w301) -> ()  [unwired: 2 in, 2 out]
            n162 = property on="Test Slider" class="Slide (strict)"("Visible"=w301) -> ()  [unwired: 2 in, 2 out]
            n163 = property on="Test Ring" class="Ring (strict)"("Visible"=w301) -> ()  [unwired: 2 in, 2 out]
            n164 = property on="Rev/Fwd" class="Clust (strict)"("Visible"=w301) -> ()  [unwired: 2 in, 2 out]
          }
          frame "Servo" {
            w317 = FALSE ("Visible")
            n165 = call <vilib>:"NT Read Number.vi"("Name"=w319) -> ("Numeric"=w318:dbl)  [unwired: 9 in, 1 out]
            n166 = property on="Test Slider" class="Slide (strict)"("Visible"=TRUE, "Scale.Maximum"=170.0 ("Scale.Range:Maximum")) -> ()  [unwired: 2 in, 2 out]
            n167 = local write "Test Slider"(w318) -> ()
            n168 = property on="Motor" class="Clust (strict)"("Visible"=w317) -> ()  [unwired: 2 in, 2 out]
            n169 = property on="Rev/Fwd" class="Clust (strict)"("Visible"=w317) -> ()  [unwired: 2 in, 2 out]
            n170 = property on="On/Off" class="Bool (strict)"("Visible"=w317) -> ()  [unwired: 2 in, 2 out]
            n171 = property on="Test Ring" class="Ring (strict)"("Visible"=w317) -> ()  [unwired: 2 in, 2 out]
          }
          frame "Relay", "Solenoid" {
            w320 = FALSE ("Visible")
            n172 = property on="Motor" class="Clust (strict)"("Visible"=w320) -> ()  [unwired: 2 in, 2 out]
            n173 = property on="Test Slider" class="Slide (strict)"("Visible"=w320) -> ()  [unwired: 2 in, 2 out]
            n174 = Search and Replace String(input string=w321, search string="/Value  **", replace string="/Direction") -> (result string=w327:string)  [unwired: 5 in, 3 out]
            n175 = property on="Test Ring" class="Ring (strict)"("Visible"=w320) -> ()  [unwired: 2 in, 2 out]
            n176 = call <vilib>:"NT Read String.vi"("Name"=w327) -> ("String"=w325:string)  [unwired: 9 in, 1 out]
            n177 = Equal?(x="Both directions", y=w325) -> (x = y?=w323:bool)
            n178 = Not(x=w323) -> (.not. x?=w324:bool)
            n179 = property on="Rev/Fwd" class="Clust (strict)"("Visible"=w323) -> ()  [unwired: 2 in, 2 out]
            n180 = property on="On/Off" class="Bool (strict)"("Visible"=w324, "Caption.Text"=w322) -> ()  [unwired: 2 in, 2 out]
          }
          frame "Compressor", "Digital Out" {
            w330 = FALSE ("Visible")
            # "Get direction and finish"
            n181 = property on="Motor" class="Clust (strict)"("Visible"=w330) -> ()  [unwired: 2 in, 2 out]
            n182 = property on="Test Slider" class="Slide (strict)"("Visible"=w330) -> ()  [unwired: 2 in, 2 out]
            n183 = property on="Test Ring" class="Ring (strict)"("Visible"=w330) -> ()  [unwired: 2 in, 2 out]
            n184 = property on="On/Off" class="Bool (strict)"("Visible"=TRUE, "Caption.Text"=w331) -> ()  [unwired: 2 in, 2 out]
            n185 = property on="Rev/Fwd" class="Clust (strict)"("Visible"=FALSE) -> ()  [unwired: 2 in, 2 out]
          }
          frame "Camera" {
            n186 = call <vilib>:"Get Last Path Segment.vi"("String in"=w338) -> ("String out"=w339:string)  [unwired: 10 in]
            n187 = property on="On/Off" class="Bool (strict)"("Visible"=FALSE) -> ()  [unwired: 2 in, 2 out]
            n188 = property on="Motor" class="Clust (strict)"("Visible"=FALSE) -> ()  [unwired: 2 in, 2 out]
            n189 = property on="Rev/Fwd" class="Clust (strict)"("Visible"=FALSE) -> ()  [unwired: 2 in, 2 out]
            n190 = case shown="\"White Balance  **\"" w339 {
              tunnel: w338 -> [w345 w354 w363 w372 w381 _ w387]
              tunnel: w337 -> [w343 w351 w360 w369 w378 _ _]
              frame "Size  **" {
                n191 = Index Array(array=w343) -> (element=w342:cluster{string[]})  [unwired: 1 in]
                n192 = call <vilib>:"NT Read String.vi"("Name"=w345) -> ("String"=w344:string)  [unwired: 9 in, 1 out]
                n193 = Unbundle(w342) -> (w340:string[])
                n194 = Match First String(2:w340, 3:w344) -> (0:w341:i32)  [unwired: 1 out]
                n195 = property on="Test Ring" class="Ring (strict)"("Value"=w341, "Strings []"=w340) -> ()  [unwired: 2 in, 2 out]
                n196 = property on="Test Ring" class="Ring (strict)"("Visible"=TRUE) -> ()  [unwired: 2 in, 2 out]
                n197 = property on="Test Slider" class="Slide (strict)"("Visible"=FALSE) -> ()  [unwired: 2 in, 2 out]
              }
              frame "White Balance  **" {
                n198 = Index Array(array=w351, index=1) -> (element=w352:cluster{string[]})
                n199 = call <vilib>:"NT Read String.vi"("Name"=w354) -> ("String"=w353:string)  [unwired: 9 in, 1 out]
                n200 = Unbundle(w352) -> (w349:string[])
                n201 = Match First String(2:w349, 3:w353) -> (0:w348:i32)  [unwired: 1 out]
                n202 = property on="Test Ring" class="Ring (strict)"("Value"=w348, "Strings []"=w349) -> ()  [unwired: 2 in, 2 out]
                n203 = property on="Test Ring" class="Ring (strict)"("Visible"=TRUE) -> ()  [unwired: 2 in, 2 out]
                n204 = property on="Test Slider" class="Slide (strict)"("Visible"=FALSE) -> ()  [unwired: 2 in, 2 out]
              }
              frame "Exposure  **" {
                n205 = Index Array(array=w360, index=2) -> (element=w361:cluster{string[]})
                n206 = call <vilib>:"NT Read String.vi"("Name"=w363) -> ("String"=w362:string)  [unwired: 9 in, 1 out]
                n207 = Unbundle(w361) -> (w357:string[])
                n208 = Match First String(2:w357, 3:w362) -> (0:w358:i32)  [unwired: 1 out]
                n209 = property on="Test Ring" class="Ring (strict)"("Value"=w358, "Strings []"=w357) -> ()  [unwired: 2 in, 2 out]
                n210 = property on="Test Ring" class="Ring (strict)"("Visible"=TRUE) -> ()  [unwired: 2 in, 2 out]
                n211 = property on="Test Slider" class="Slide (strict)"("Visible"=FALSE) -> ()  [unwired: 2 in, 2 out]
              }
              frame "Exposure Priority  **" {
                n212 = Index Array(array=w369, index=3) -> (element=w370:cluster{string[]})
                n213 = call <vilib>:"NT Read String.vi"("Name"=w372) -> ("String"=w371:string)  [unwired: 9 in, 1 out]
                n214 = Unbundle(w370) -> (w366:string[])
                n215 = Match First String(2:w366, 3:w371) -> (0:w367:i32)  [unwired: 1 out]
                n216 = property on="Test Ring" class="Ring (strict)"("Value"=w367, "Strings []"=w366) -> ()  [unwired: 2 in, 2 out]
                n217 = property on="Test Ring" class="Ring (strict)"("Visible"=TRUE) -> ()  [unwired: 2 in, 2 out]
                n218 = property on="Test Slider" class="Slide (strict)"("Visible"=FALSE) -> ()  [unwired: 2 in, 2 out]
              }
              frame "Color Enable  **" {
                n219 = Index Array(array=w378, index=4) -> (element=w379:cluster{string[]})
                n220 = call <vilib>:"NT Read String.vi"("Name"=w381) -> ("String"=w380:string)  [unwired: 9 in, 1 out]
                n221 = Unbundle(w379) -> (w375:string[])
                n222 = Match First String(2:w375, 3:w380) -> (0:w376:i32)  [unwired: 1 out]
                n223 = property on="Test Ring" class="Ring (strict)"("Value"=w376, "Strings []"=w375) -> ()  [unwired: 2 in, 2 out]
                n224 = property on="Test Ring" class="Ring (strict)"("Visible"=TRUE) -> ()  [unwired: 2 in, 2 out]
                n225 = property on="Test Slider" class="Slide (strict)"("Visible"=FALSE) -> ()  [unwired: 2 in, 2 out]
              }
              frame Default {
                n226 = property on="Test Ring" class="Ring (strict)"("Visible"=FALSE) -> ()  [unwired: 2 in, 2 out]
                n227 = property on="Test Slider" class="Slide (strict)"("Visible"=FALSE) -> ()  [unwired: 2 in, 2 out]
              }
              frame "Brightness  **", "Color Level  **", "Compression  **", "FPS  **", "Sharpness  **" {
                n228 = call <vilib>:"NT Read Number.vi"("Name"=w387) -> ("Numeric"=w386:dbl)  [unwired: 9 in, 1 out]
                n229 = local write "Test Slider"(w386) -> ()
                n230 = property on="Test Slider" class="Slide (strict)"("Visible"=TRUE, "Scale.Maximum"=100.0 ("Scale.Range:Maximum")) -> ()  [unwired: 2 in, 2 out]
                n231 = property on="Test Ring" class="Ring (strict)"("Visible"=FALSE) -> ()  [unwired: 2 in, 2 out]
              }
            }
          }
        }
        n232 = property on="Progress" class="Clust (strict)"("Visible"=FALSE) -> ()  [unwired: 2 in, 2 out]
      }
      event "Test Name": Mouse Enter {
        # "Populate the ring with the list of tests"
        n233 = event-data() -> ()  [unwired: 1 in, 1 out]
        n234 = call <vilib>:"NT Read String Array.vi"("Name"="/TestMode/TestList") -> ("String Array"=w395:string[])  [unwired: 9 in, 1 out]
        n235 = Build Array (concatenate)("Select the test to run...", w395) -> (w394:string[])
        n236 = property on="Test Name" class="Ring (strict)"("Strings []"=w394) -> ()  [unwired: 2 in, 2 out]
      }
      event "Test Name": Value Change {
        w397 = FALSE ("Visible")
        # "Tell the robot the test name to run"
        n237 = event-data() -> ("NewVal"=w401:u16)  [unwired: 1 in]
        n238 = property on="Test Name" class="Ring (strict)"() -> ("Strings []"=w402:string[])  [unwired: 2 in, 2 out]
        n239 = local write "Progress"(T6 {"Test Progress"=0, "Test Progress Text"=""} ("Progress")) -> ()
        n240 = Index Array(array=w402, index=w401) -> (element=w400:string)
        n241 = call <vilib>:"NT Write String.vi"("String"=w400, "Name"="/TestMode/TestName") -> ()  [unwired: 9 in, 1 out]
        n242 = property on="Progress" class="Clust (strict)"("Visible"=TRUE) -> ()  [unwired: 2 in, 2 out]
        n243 = property on="Motor" class="Clust (strict)"("Visible"=w397) -> ()  [unwired: 2 in, 2 out]
        n244 = property on="Test Slider" class="Slide (strict)"("Visible"=w397) -> ()  [unwired: 2 in, 2 out]
        n245 = property on="On/Off" class="Bool (strict)"("Visible"=w397) -> ()  [unwired: 2 in, 2 out]
        n246 = property on="Rev/Fwd" class="Clust (strict)"("Visible"=w397) -> ()  [unwired: 2 in, 2 out]
        n247 = property on="Test Ring" class="Ring (strict)"("Visible"=w397) -> ()  [unwired: 2 in, 2 out]
      }
      event "Select Auto": Mouse Enter {
        # "Populate the combo box with the list of autonomous options"
        n248 = event-data() -> ()  [unwired: 1 in, 1 out]
        n249 = call <vilib>:"NT Read String Array.vi"("Name"="Auto List") -> ("String Array"=w404:string[])  [unwired: 9 in, 1 out]
        n250 = property on="Select Auto" class="CmbBox"("Strings[]"=w404) -> ()  [unwired: 2 in, 2 out]
      }
      event "Select Auto": Value Change {
        # "User modified the Auto Selection. Write to NT variable so robot knows."
        n251 = event-data() -> ("NewVal"=w407:string)  [unwired: 1 in]
        n252 = call <vilib>:"NT Write String.vi"("String"=w407, "Name"="Auto Selector") -> ()  [unwired: 9 in, 1 out]
      }
      event "Command Selection": Value Change {
        # "Get the params and show in table"
        n253 = event-data() -> ("NewVal"=w413:i32)  [unwired: 1 in]
        n254 = property on="Command Selection" class="MCListbox (strict)"() -> ("ItemNames"=w411:string[][])  [unwired: 2 in, 2 out]
        n255 = call <vilib>:"WPI_DashboardUpdate Command Params.vi"("NewVal"=w413, "Commands"=w411, "Param Tbl"=w412) -> ()  [unwired: 8 in, 1 out]
      }
      event "Execute Command": Value Change {
        # "Started one, Unique ID holds\nresponse"
        n256 = event-data() -> ()  [unwired: 1 in, 1 out]
        n257 = property on="Command Selection" class="MCListbox (strict)"() -> ("ItemNames"=w424:string[][])  [unwired: 2 in, 2 out]
        n258 = Index Array(array=w424, index (row)="Command Selection", index (col)=0) -> (element=w422:string)
        n259 = call <vilib>:"Invoke Commands.vi"("Command Params"="Command Params", "Function Name"=w422) -> ("Params"=w418:u8, "Started"=w417:bool)  [unwired: 7 in, 1 out]
        n260 = Array Subset(array="Command Params", length (row)=w418) -> (w419:string[][])  [unwired: 3 in]
        n261 = Select(t="Executing" ("Cmd Status"), s=w417, f="" ("Cmd Status")) -> (s? t:f=→"Cmd Status":string)
      }
      event "Command Selection": Double Click {
        n262 = event-data() -> ("Row"=w432:i32)  [unwired: 1 in]
        n263 = property on="Command Selection" class="MCListbox (strict)"() -> ("ItemNames"=w435:string[][])  [unwired: 2 in, 2 out]
        n264 = local read "Command Params"() -> (w431:string[][])
        n265 = Index Array(array=w435, index (row)=w432, index (col)=0) -> (element=w433:string)
        n266 = call <vilib>:"Invoke Commands.vi"("Command Params"=w431, "Function Name"=w433) -> ("Params"=w430:u8, "Started"=w425:bool)  [unwired: 7 in, 1 out]
        n267 = Array Subset(array=w431, length (row)=w430) -> (w429:string[][])  [unwired: 3 in]
        n268 = Select(t="Executing" ("Cmd Status"), s=w425, f="" ("Cmd Status")) -> (s? t:f=w426:string)
        n269 = local write "Cmd Status"(w426) -> ()
      }
      event "CheckList": Double Click {
        # "Shift clears all"
        # "Update symbols on the listbox"
        n270 = event-data() -> ("PlatMods.Shift"=w437:bool, "Row"=w439:i32)  [unwired: 1 in]
        n271 = case shown="True" w437 {
          tunnel: w439 -> [w443 _]
          tunnel: 1 -> [w442 _]
          frame False {
            n272 = property on="CheckList" class="LstBox (strict)"() -> ("Item Symbols"=w441:i32[])  [unwired: 2 in, 2 out]
            n273 = Replace Array Subset(array=w441, new element=w442, index=w443) -> (w440:i32[])
            n274 = property on="CheckList" class="LstBox (strict)"("Item Symbols"=w440) -> ()  [unwired: 2 in, 2 out]
          }
          frame True {
            w444 = 0 ("Top Row")
            n275 = property on="CheckList" class="LstBox (strict)"() -> ("Number of Rows"=w446:u32)  [unwired: 2 in, 2 out]
            n276 = Initialize Array(0, w446) -> (w445:i32[])
            n277 = property on="CheckList" class="LstBox (strict)"("Top Row"=w444, "Value"=w444, "Item Symbols"=w445) -> ()  [unwired: 2 in, 2 out]
          }
        }
      }
      event "CheckList": Key Down {
        # "Update symbols on the listbox\nLeft and right keys check and uncheck"
        n278 = event-data() -> ("VKey"=w450:T18)  [unwired: 1 in]
        n279 = case shown="\"Left\", \"Right\"" w450 {
          selector: w450 -> [w455 _]
          tunnel: eventvkey."Left" ("VKey") -> [w453 _]
          frame "Left", "Right" {
            n280 = Equal?(x=w453, y=w455) -> (x = y?=w454:bool)
            n281 = Select(t=0, s=w454, f=1) -> (s? t:f=w456:i32)
            n282 = property on="CheckList" class="LstBox (strict)"() -> ("Item Symbols"=w459:i32[])  [unwired: 2 in, 2 out]
            n283 = Replace Array Subset(array=w459, new element=w456, index="CheckList") -> (w458:i32[])
            n284 = property on="CheckList" class="LstBox (strict)"("Item Symbols"=w458) -> ()  [unwired: 2 in, 2 out]
          }
          frame Default {
          }
        }
      }
      event "Motor.Enable": Value Change {
        # "When the test mode otor enable helper is set, update that\ntree row item's value"
        n285 = event-data() -> ("NewVal"=w465:bool)  [unwired: 1 in]
        n286 = Unbundle("Motor") -> ("Value"=w464:dbl)  [unwired: 1 out]
        n287 = Select(t=w464, s=w465, f=0.0) -> (s? t:f=w462:dbl)
        n288 = call <vilib>:"NT Write Number.vi"("Numeric"=w462, "Name"=w461) -> ()  [unwired: 9 in, 1 out]
      }
      event "Test Slider": Value Change {
        # "When the test mode slider helper is set, update that\ntree row item's value"
        n289 = event-data() -> ("NewVal"=w468:dbl)  [unwired: 1 in]
        n290 = call <vilib>:"NT Write Number.vi"("Numeric"=w468, "Name"=w469) -> ()  [unwired: 9 in, 1 out]
      }
      event "On/Off": Value Change {
        # "When the test mode on/off helper value is set, update that\ntree row item's value"
        n291 = event-data() -> ("NewVal"=w473:bool)  [unwired: 1 in]
        n292 = Boolean To (0,1)(Boolean=w473) -> (0, 1=w472:i16)
        n293 = call <vilib>:"NT Write Number.vi"("Numeric"=w472, "Name"=w471) -> ()  [unwired: 9 in, 1 out]
      }
      event "Rev/Fwd": Value Change {
        # "When the test mode helper value for relays is set, update that\ntree row item's value"
        n294 = event-data() -> ("NewVal.Forward"=w481:bool, "NewVal.Reverse"=w480:bool)  [unwired: 1 in]
        n295 = Boolean To (0,1)(Boolean=w481) -> (0, 1=w477:i16)
        n296 = Boolean To (0,1)(Boolean=w480) -> (0, 1=w479:i16)
        n297 = Negate(x=w479) -> (-x=w478:i16)
        n298 = Add(x=w477, y=w478) -> (x+y=w476:i16)
        n299 = call <vilib>:"NT Write Number.vi"("Numeric"=w476, "Name"=w475) -> ()  [unwired: 9 in, 1 out]
      }
      event "Test Ring": Value Change {
        # "When a test mode helper value is selected from the ring,\nset the tree item's variable to the string value"
        n300 = event-data() -> ("NewVal"=w485:u16)  [unwired: 1 in]
        n301 = property on="Test Ring" class="Ring (strict)"() -> ("Strings []"=w486:string[])  [unwired: 2 in, 2 out]
        n302 = Index Array(array=w486, index=w485) -> (element=w484:string)
        n303 = call <vilib>:"NT Write String.vi"("String"=w484, "Name"=w483) -> ()  [unwired: 9 in, 1 out]
      }
      event "Rec Mode": Value Change {
        # "Update globals for recording mode and path to read log from.\nClear when logging and let NetworkTables set path for vision to\nuse."
        n304 = event-data() -> ("NewVal"=w497:enum32{"Stop", "Record", "Playback"})  [unwired: 1 in]
        n305 = global write "WPI_DashboardLogging Global.vi" "Logging Filename"(path "") -> ()
        n306 = global write "WPI_DashboardLogging Global.vi" "Recording"(w497) -> ()
        n307 = case shown="\"Playback\"" w497 {
          tunnel: w496 -> [_ w499 w508]
          tunnel: [_ _ w507] -> w494
          tunnel: [_ _ w506] -> _
          tunnel: w492 -> [_ _ w504]
          tunnel: cluster{i32, i32} {-250, 170} -> [_ _ w503]
          tunnel: [_ _ T19 {"Image Size"=TRUE, "Image Type"=TRUE, "Pixel Value"=TRUE, "ROI Information"=TRUE, "Zoom Factor"=FALSE} ("Image Information Shown:All Elements")] -> w490
          tunnel: [_ _ TRUE ("Zoom Factor")] -> w489
          tunnel: w488 -> [_ _ w500]
          frame Default {
          }
          frame "Stop", "Record" {
            # "Place Window too"
            n308 = invoke class="VI" method="FP.Close"(reference=w499) -> (reference out=w498:refnum<vi>)  [unwired: 2 in, 2 out]
            n309 = invoke class="VI" method="Abort VI"(reference=w498) -> ()  [unwired: 2 in, 3 out]
          }
          frame "Playback" {
            n310 = call "Open Playback Panel.vi"("Offset"=w503, "DB VI Ref"=w504, "Playback in"=w508) -> ("Playback out"=w505:refnum<vi>)  [unwired: 8 in]
            n311 = register-events(w505, w500) -> (reference out=w507:refnum<event-registration>, error out=w506:errorcluster)  [unwired: 2 in]
          }
        }
        n312 = property on="Camera Image" class="ImageControl"("Image Information Shown"=w490, "Image Information Visible"=w489) -> ()  [unwired: 2 in, 2 out]
        n313 = call <vilib>:"WPI_DashboardNT Log FieldName Cache.vi"("Operation"=enum16{"Lookup/Add", "Index", "Clear"}."Clear") -> ()  [unwired: 8 in, 3 out]
      }
      event Panel Close {
        w510 = enum32{"Stop", "Record", "Playback"}."Stop" ("Rec Mode")
        # "Playback window has been closed, abort"
        n314 = event-data() -> ()  [unwired: 1 in, 4 out]
        n315 = local write "Rec Mode"(w510) -> ()
        n316 = global write "WPI_DashboardLogging Global.vi" "Recording"(w510) -> ()
      }
      event Panel Close {
        # "Abort playback window and ourself"
        n317 = event-data() -> ()  [unwired: 1 in, 4 out]
        n318 = invoke class="VI" method="FP.Close"(reference=w514) -> (reference out=w513:refnum<vi>)  [unwired: 2 in, 2 out]
        n319 = invoke class="VI" method="Abort VI"(reference=w513) -> (error out=w512:errorcluster)  [unwired: 2 in, 2 out]
        n320 = invoke class="VI" method="Abort VI"(error in=w512) -> ()  [unwired: 2 in, 3 out]
      }
      event User Event {
        n321 = event-data() -> ("IDs"=w521:cluster{"RPC field ID":u16, "Unique ID":u16}, "String"=w520:string)  [unwired: 1 in]
        n322 = Bundle("IDs"=w521, "String"=w520) -> (w519:T8)  [unwired: 1 in]
        n323 = call <vilib>:"Retrieve RPC Response.vi"("RPC Response"=w519) -> ("Output"=w517:string[][])  [unwired: 10 in]
        n324 = Build Array (concatenate)(w515, w517) -> (w516:string[][])
        n325 = local write "Command Params"(w516) -> ()
        n326 = local write "Cmd Status"("" ("Cmd Status")) -> ()
      }
      event "Tree": Double Click {
        n327 = event-data() -> ("PlatMods"=w525:T22, "Tag"=w524:string)  [unwired: 1 in]
        n328 = Unbundle(w525) -> ("Shift"=w523:bool)  [unwired: 4 out]
        n329 = Not(x=w523) -> (.not. x?=w522:bool)
        n330 = call <vilib>:"NT Update Persistence.vi"("Persistence"=w522, "Name"=w524) -> ()  [unwired: 9 in, 1 out]
      }
    }
  }
  n331 = while {
    tunnel: w62 -> [w528]
    i -> [w531]
    stop <- FALSE stop-if-true
    n332 = Wait (ms)(milliseconds to wait=u32 100) -> ()  [unwired: 1 out]
    n333 = case shown="\"Playback\"" "Rec Mode" {
      tunnel: w531 -> [_ _ w546]
      tunnel: [u32 2829099 ("Base Color") u32 11141120 ("Target Color") w535] -> w527
      frame "Stop", Default {
        # "Reset the color, extra updates don't cost much"
      }
      frame "Record" {
      }
      frame "Playback" {
        # "Playback"
        n334 = Quotient & Remainder(x=w546, y=u32 50 ("milliseconds to wait")) -> (x-y*floor(x/y)=w542:u32)  [unwired: 1 out]
        n335 = Divide(x=w542, y=u32 50 ("milliseconds to wait")) -> (x/y=w539:dbl)
        n336 = Multiply(x=6.283185307179586, y=w539) -> (x*y=w544:dbl)
        n337 = Sine(x=w544) -> (sin(x)=w543:dbl)
        n338 = Absolute Value(x=w543) -> (abs(x)=w536:dbl)
        n339 = call "Interpolate RGB Color.vi"("Proportion"=w536, "Target Color"=u32 30976, "Base Color"=u32 2829099) -> ("Result Color"=w535:u32)  [unwired: 8 in]
      }
    }
    n340 = property class="Pane"(reference=w528, "PaneColor"=w527) -> ()  [unwired: 1 in, 2 out]
  }
  n341 = local write "Dashboard Tab"(T2."Drive" ("Dashboard Tab")) -> ()
  n342 = property on="On/Off" class="Bool (strict)"("Visible"=w33) -> ()  [unwired: 2 in, 2 out]
  n343 = property on="Motor" class="Clust (strict)"("Visible"=w33) -> ()  [unwired: 2 in, 2 out]
  n344 = property on="Progress" class="Clust (strict)"("Visible"=w33) -> ()  [unwired: 2 in, 2 out]
  n345 = property on="Test Ring" class="Ring (strict)"("Visible"=w33) -> ()  [unwired: 2 in, 2 out]
  n346 = property on="Rev/Fwd" class="Clust (strict)"("Visible"=w33) -> ()  [unwired: 2 in, 2 out]
  n347 = while {
    tunnel: u16 1741 ("timeout ms (25000)") -> [w548]
    stop <- FALSE stop-if-true
    n348 = TCP Create Listener(10:w548) -> (0:w547:errorcluster, 3:w549:refnum<k5>)  [unwired: 4 in, 1 out]
    n349 = case shown="No Error" w547 {
      selector: w547 -> [w551 _]
      tunnel: w549 -> [w552 _]
      frame No Error {
        n350 = while {
          tunnel: w552 -> [w555]
          tunnel: w551 -> [w554]
          stop <- FALSE stop-if-true
          n351 = TCP Wait On Listener(8:w554, 11:w555) -> (0:w556:errorcluster, 4:w557:refnum<k5>)  [unwired: 2 in, 3 out]
          n352 = local write "TCP"(w557) -> ()
          n353 = case shown="No Error" w556 {
            frame No Error {
            }
            frame Error {
              n354 = Wait (ms)(milliseconds to wait=u32 1000) -> ()  [unwired: 1 out]
            }
          }
        }
      }
      frame Error {
        n355 = Wait (ms)(milliseconds to wait=u32 1000) -> ()  [unwired: 1 out]
      }
    }
  }
  n356 = local write "Command Selection"(u16 0 ("milliseconds to wait")) -> ()
  n357 = local write "Command Params"(string[][] [] ("Command Params")) -> ()
  n358 = global write "WPI_DashboardLogging Global.vi" "Recording"(w56) -> ()
  n359 = local write "Rec Mode"(w56) -> ()
  n360 = call <vilib>:"NT Write String.vi"("String"="Select Auto", "Name"="Auto Selector") -> ()  [unwired: 9 in, 1 out]
